vi "Main.vi"() -> (0 "error out":errorcluster)   [LabVIEW 2018]
uses:
  Controls/Cluster_HMI_VIFP - 2.ctl
  <vilib>/RAFA Solutions/Harmony UI Controls Kit/Numeric/Horizontal Progress Bar.ctl
  <vilib>/RAFA Solutions/Harmony UI Controls Kit/Numeric/Numeric Indicator.ctl
  Global/Demo.vi
  Global/Error Queue Reference.vi
  Global/datos usuario.vi
  <vilib>/addons/database/Connection.llb/DB Tools Open Connec (Path).vi
  Global/TimerReferences.vi
  Global/globalGenerador2_HMI.vi
  Global/globalGenerador3_HMI.vi
  Global/globalGenerador4_HMI.vi
  Global/globalGenerador5_HMI.vi
  Global/globalGenerador6_HMI.vi
  Global/globalGenerador1_HMI.vi
  Global/globalEventos.vi
  Global/MSG.vi
  <vilib>/addons/database/NI_Database_API.lvlib
  <vilib>/RAFA Solutions/Harmony UI Controls Kit/Flat UI Design.lvlib
panel:
  in  "type specifier VI Refnum (for type only) 16":refnum<vi>
  out "Mensaje Error":string
  in  "type specifier VI Refnum (for type only)":refnum<vi>
  in  "type specifier VI Refnum (for type only) 15":refnum<vi>
  in  "type specifier VI Refnum (for type only) 14":refnum<vi>
  in  "type specifier VI Refnum (for type only) 13":refnum<vi>
  in  "type specifier VI Refnum (for type only) 12":refnum<vi>
  in  "type specifier VI Refnum (for type only) 11":refnum<vi>
  in  "type specifier VI Refnum (for type only) 10":refnum<vi>
  in  "type specifier VI Refnum (for type only) 9":refnum<vi>
  in  "type specifier VI Refnum (for type only) 8":refnum<vi>
  in  "type specifier VI Refnum (for type only) 7":refnum<vi>
  in  "type specifier VI Refnum (for type only) 6":refnum<vi>
  in  "type specifier VI Refnum (for type only) 5":refnum<vi>
  in  "type specifier VI Refnum (for type only) 4":refnum<vi>
  in  "type specifier VI Refnum (for type only) 3":refnum<vi>
  in  "type specifier VI Refnum (for type only) 2":refnum<vi>
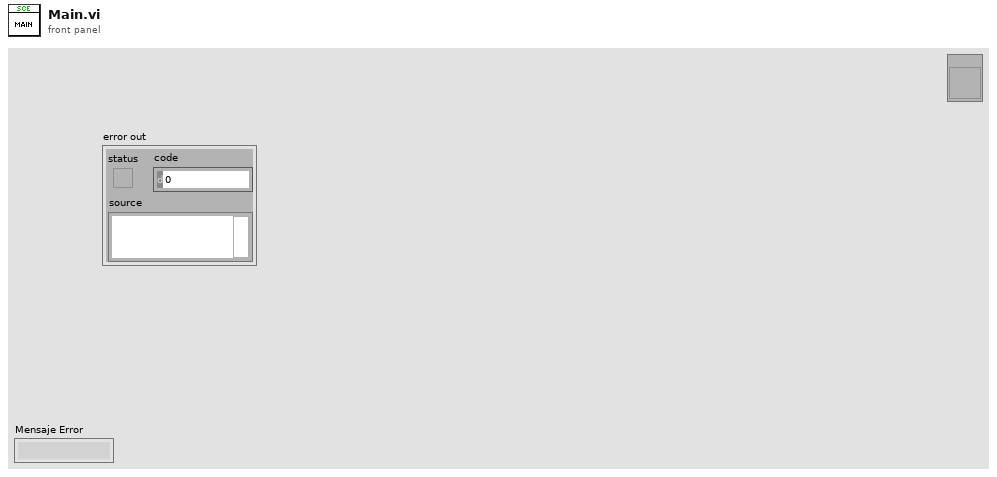
[diagram p1: front panel]
types:
  T1 = enum32{"Invalid", "Standard", "Closed", "Hidden", "Minimized", "Maximized"}
  T2 = typedef "NI_Database_API.lvlib/Conn ObjectReference.ctl" = refnum<k1>
  T3 = typedef "Equipos_Medicion_cluster.ctl" = cluster{"ID_EQUIPO":i32, "IP_EQUIPO":string, "NOMBRE_EQUIPO":string, "ESTADO_EQUIPO":string, "DESCRIPCION":string, "ID_MEDICION":i32, "ESTADO_MEDICION":string, "TIEMPO_MEDICION":string}
  T4 = typedef "Cluster_HMI_VIFP - 2.ctl" = cluster{"L2":T5, "L3":T5, "I2":T5, "I3":T5, "Frecuencia [Hz]":T6, "Potencia Total [kW]":T6, "Factor de Potencia":T6, "L1":T5, "I1":T5}
  T5 = typedef "Flat UI Design.lvlib/Horizontal Progress Bar.ctl" = sgl
  T6 = typedef "Flat UI Design.lvlib/Numeric Indicator.ctl" = sgl
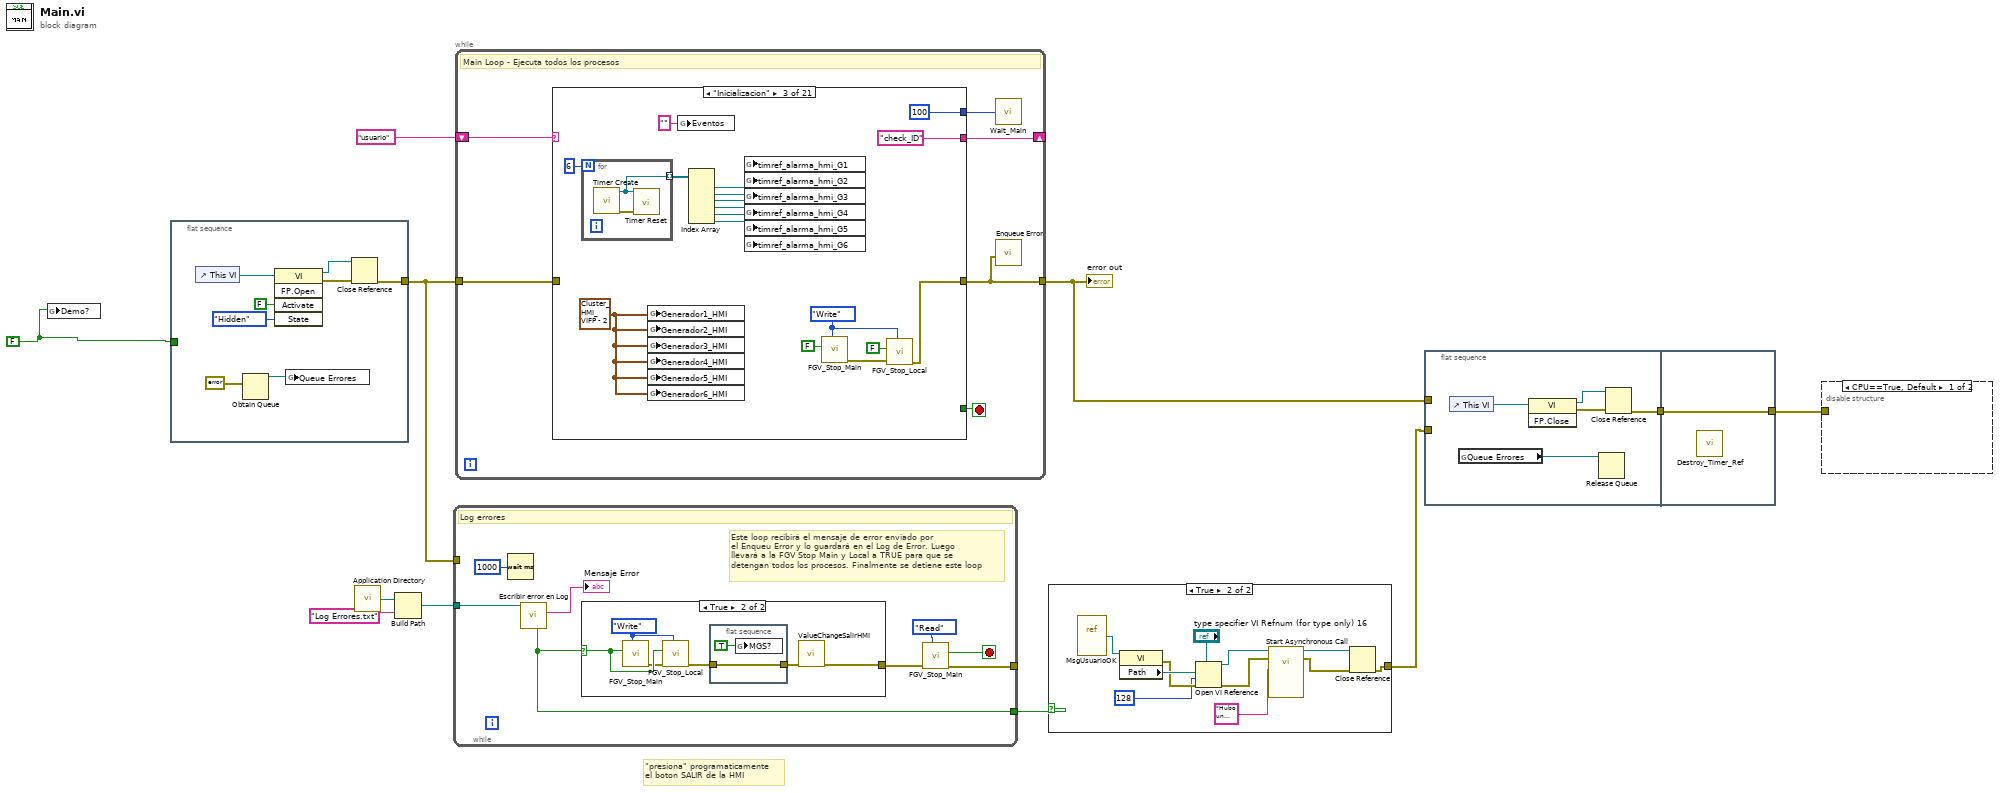
[diagram p0: block diagram]
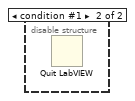
[diagram p4: hidden frame]
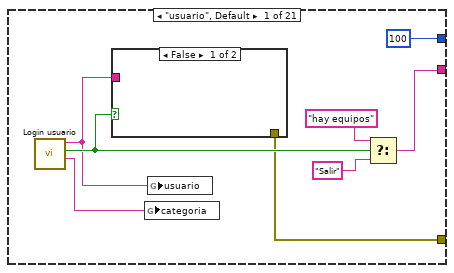
[diagram p5: hidden frame]
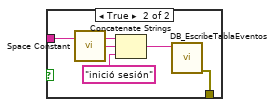
[diagram p6: hidden frame]
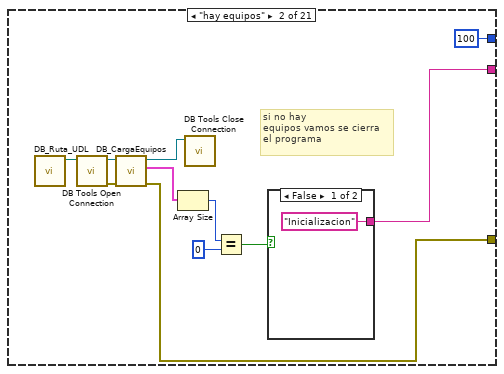
[diagram p7: hidden frame]
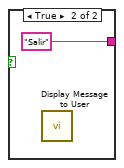
[diagram p8: hidden frame]
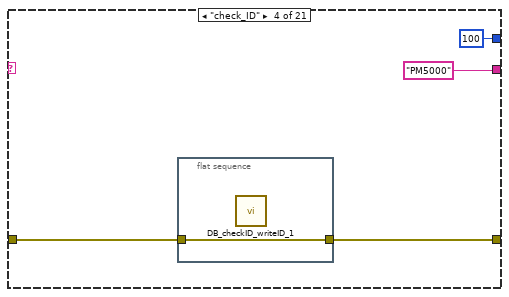
[diagram p9: hidden frame]
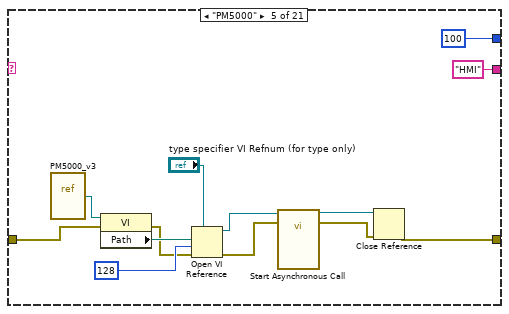
[diagram p10: hidden frame]
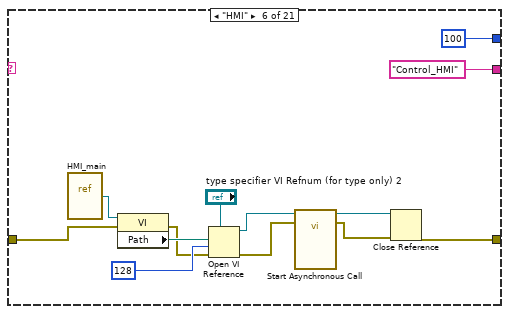
[diagram p11: hidden frame]
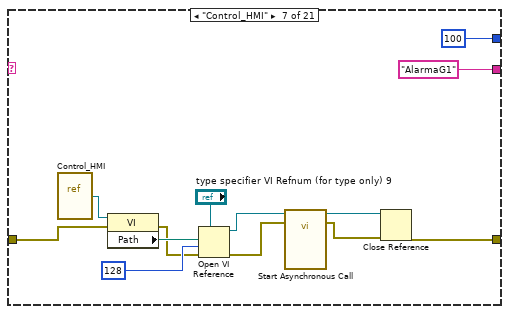
[diagram p12: hidden frame]
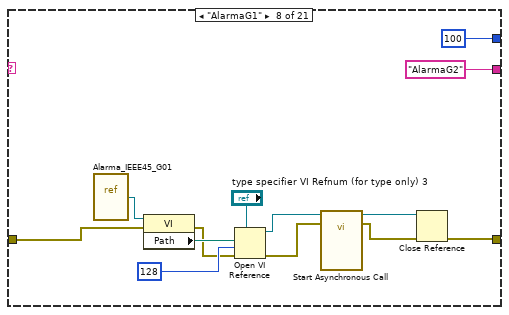
[diagram p13: hidden frame]
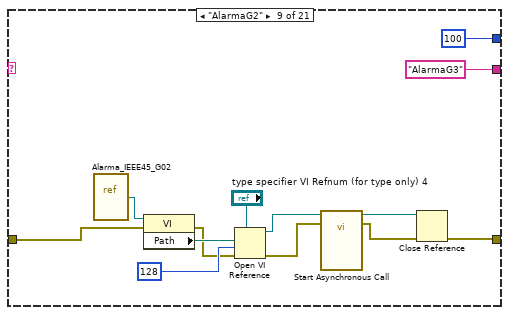
[diagram p14: hidden frame]
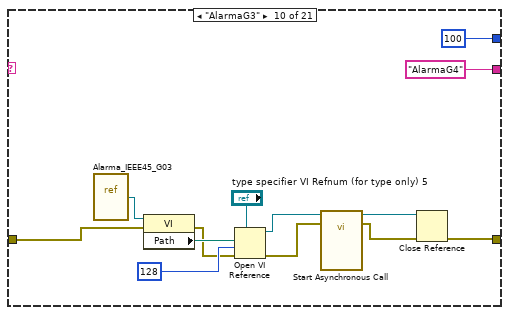
[diagram p15: hidden frame]
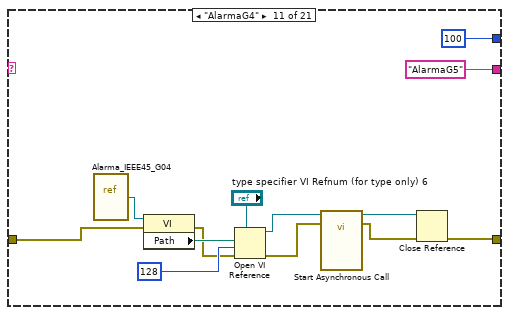
[diagram p16: hidden frame]
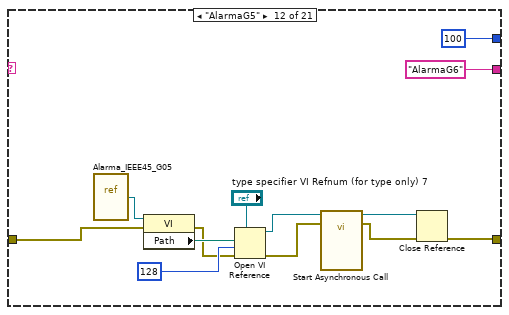
[diagram p17: hidden frame]
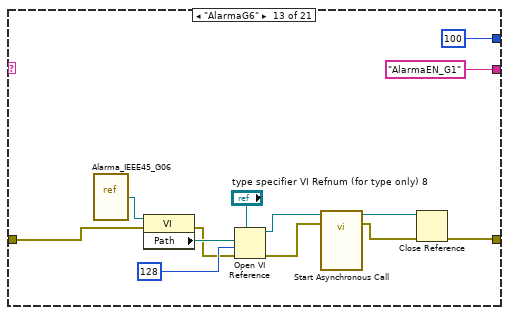
[diagram p18: hidden frame]
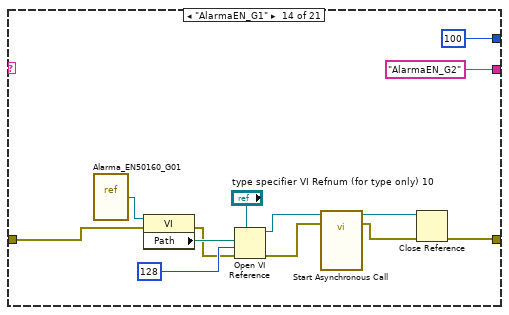
[diagram p19: hidden frame]
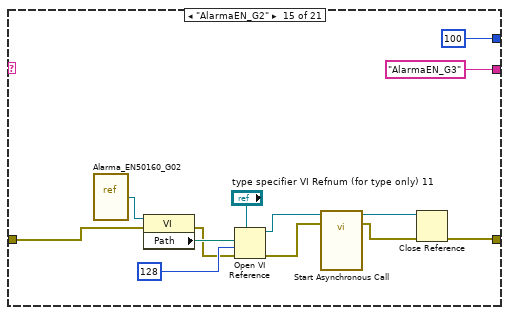
[diagram p20: hidden frame]
diagram:
  w2 = FALSE ("Demo?")
  # "\"presiona\" programaticamente\nel boton SALIR de la HMI"
  n1 = global write "Demo.vi" "Demo?"(w2) -> ()
  n2 = flat-sequence {
    tunnel: [w14] -> w7
    tunnel: w2 -> [_]
    frame #0 {
      n3 = control-ref of="This VI"() -> (w19:refnum<vi>)
      n4 = Obtain Queue(element data type=errorcluster {"status"=FALSE, "code"=0, "source"=""} ("error out")) -> (queue out=w13:refnum<queue>)  [unwired: 4 in, 2 out]
      n5 = invoke class="VI" method="FP.Open"(reference=w19, "Activate"=FALSE ("Activate?"), "State"=T1."Hidden") -> (reference out=w16:refnum<vi>, error out=w15:errorcluster)  [unwired: 2 in, 3 out]
      n6 = global write "Error Queue Reference.vi" "Queue Errores"(w13) -> ()
      n7 = Close Reference(reference=w16, error in (no error)=w15) -> (error out=w14:errorcluster)
    }
  }
  n8 = call <vilib>:"Application Directory.vi"() -> ("Application Directory"=w10:path)
  n9 = Build Path(base path=w10, name or relative path="Log Errores.txt") -> (appended path=w8:path)
  n10 = while {
    tunnel: w8 -> [w27]
    tunnel: w7 -> [_]
    tunnel: [w22] -> _
    tunnel: [w20] -> w6
    stop <- w23 stop-if-true
    # "Este loop recibirá el mensaje de error enviado por \nel Enqueu Error y lo guardará en el Log de Error. Luego\nllevará a la FGV Stop Main y Local a TRUE para que se\ndetengan todos los procesos. Finalmente se detiene este loop"
    # "Log errores"
    n11 = Wait (ms)(milliseconds to wait=u32 1000) -> ()  [unwired: 1 out]
    n12 = call "Escribir error en Log.vi"("Ruta Log"=w27) -> ("Mensaje Error"=→"Mensaje Error":string, "error"=w20:bool)  [unwired: 6 in, 3 out]
    n13 = case shown="True" w20 {
      selector: w20 -> [_ w32]
      tunnel: [_ w28] -> w21
      frame False {
      }
      frame True {
        w33 = enum16{"Read", "Write"}."Write" ("Action")
        n14 = call "FGV_Stop_Main.vi"("Action"=w33, "Var In"=w32) -> ("Error Out"=w31:errorcluster)  [unwired: 8 in, 1 out]
        n15 = call "FGV_Stop_Local.vi"("Action"=w33, "Error In (no error)"=w31, "Var In"=w32) -> ("Error Out"=w30:errorcluster)  [unwired: 7 in, 1 out]
        n16 = flat-sequence {
          tunnel: w30 -> [w34]
          tunnel: [w34] -> w29
          frame #0 {
            n17 = global write "MSG.vi" "MGS?"(TRUE ("MGS?")) -> ()
          }
        }
        n18 = call "ValueChangeSalirHMI.vi"("error in (no error)"=w29) -> ("error out"=w28:errorcluster)  [unwired: 10 in]
      }
    }
    n19 = call "FGV_Stop_Main.vi"("Action"=enum16{"Read", "Write"}."Read", "Error In (no error)"=w21) -> ("Error Out"=w22:errorcluster, "Var Out"=w23:bool)  [unwired: 8 in]
  }
  n20 = while {
    shift-right: [w40] -> _
    shift-left: "usuario" -> [w41]
    tunnel: w7 -> [w37]
    tunnel: [w36] -> w5
    stop <- w39 stop-if-true
    # "Main Loop - Ejecuta todos los procesos"
    n21 = case shown="\"Inicializacion\"" w41 {
      tunnel: [w46 w61 "check_ID" "PM5000" "HMI" "Control_HMI" "AlarmaG1" "AlarmaG2" "AlarmaG3" "AlarmaG4" "AlarmaG5" "AlarmaG6" "AlarmaEN_G1" "AlarmaEN_G2" "AlarmaEN_G3" "AlarmaEN_G4" "AlarmaEN_G5" "AlarmaEN_G6" "Idle" w289 ""] -> w40
      tunnel: [_ _ _ _ _ _ _ _ _ _ _ _ _ _ _ _ _ _ _ _ TRUE] -> w39
      tunnel: [u32 100 ("Wait time (msec)") u32 100 ("Wait time (msec)") u32 100 ("Wait time (msec)") u32 100 ("Wait time (msec)") u32 100 ("Wait time (msec)") u32 100 ("Wait time (msec)") u32 100 ("Wait time (msec)") u32 100 ("Wait time (msec)") u32 100 ("Wait time (msec)") u32 100 ("Wait time (msec)") u32 100 ("Wait time (msec)") u32 100 ("Wait time (msec)") u32 100 ("Wait time (msec)") u32 100 ("Wait time (msec)") u32 100 ("Wait time (msec)") u32 100 ("Wait time (msec)") u32 100 ("Wait time (msec)") u32 100 ("Wait time (msec)") u32 100 ("Wait time (msec)") u32 1000 ("Wait time (msec)") u32 100 ("Wait time (msec)")] -> w38
      tunnel: w37 -> [_ _ _ w88 w95 w106 w121 w132 w145 w158 w171 w184 w197 w210 w223 w236 w249 w262 w275 _ w294]
      tunnel: [w42 w56 w69 w87 w103 w105 w120 w131 w144 w157 w170 w183 w196 w209 w222 w235 w248 w261 w274 w287 w294] -> w36
      frame "usuario", Default {
        n22 = call "Login usuario.vi"() -> ("categoria out"=w43:string, "Usuario y Pass OK?"=w45:bool, "Usuario out"=w44:string)  [unwired: 9 in]
        n23 = case shown="False" w45 {
          tunnel: w44 -> [_ w54]
          tunnel: [_ w50] -> w42
          frame False {
          }
          frame True {
            n24 = call <vilib>:"Space Constant.vi"() -> ("String"=w53:string)
            n25 = Concatenate Strings(w54, w53, "inició sesión" ("string")) -> (w51:string)
            n26 = call "DB_EscribeTablaEventos.vi"("DESCRIPCION"=w51) -> ("error out"=w50:errorcluster)  [unwired: 10 in]
          }
        }
        n27 = global write "datos usuario.vi" "categoria"(w43) -> ()
        n28 = global write "datos usuario.vi" "usuario"(w44) -> ()
        n29 = Select(t="hay equipos", s=w45, f="Salir") -> (s? t:f=w46:string)
      }
      frame "hay equipos" {
        # "si no hay \nequipos vamos se cierra \nel programa"
        n30 = call "DB_Ruta_UDL.vi"() -> ("UDL ruta"=w57:path)  [unwired: 11 in]
        n31 = call-poly <vilib>:"DB Tools Open Connection.vi"("connection information"=w57) -> ("error out"=w59:errorcluster, "connection reference"=w58:T2)  [unwired: 7 in]
        n32 = call "DB_CargaEquipos.vi"("error in (no error)"=w59, "db in"=w58) -> ("error out"=w56:errorcluster, "Equipos_out"=w63:T3[], "db out"=w55:T2)  [unwired: 2 in, 5 out]
        n33 = Array Size(array=w63) -> (size(s)=w65:i32)
        n34 = call <vilib>:"DB Tools Close Connection.vi"("connection reference"=w55) -> ()  [unwired: 6 in, 1 out]
        n35 = Equal?(x=w65, y=0) -> (x = y?=w62:bool)
        n36 = case shown="False" w62 {
          tunnel: ["Inicializacion" "Salir"] -> w61
          frame False {
          }
          frame True {
            n37 = call "Display Message to User"() -> ()  [unwired: 10 in, 2 out]
          }
        }
      }
      frame "Inicializacion" {
        w70 = T4 {"L2"=0.0, "L3"=0.0, "I2"=0.0, "I3"=0.0, "Frecuencia [Hz]"=0.0, "Potencia Total [kW]"=0.0, "Factor de Potencia"=0.0, "L1"=0.0, "I1"=0.0} ("Generador1_HMI")
        w81 = enum16{"Read", "Write"}."Write" ("Action")
        n38 = for {
          N: 6 -> [_]
          tunnel: [w85] -> w78 mode=indexing
          n39 = call "Timer Create.vi"() -> ("error out"=w86:errorcluster, "Timer reference out"=w85:refnum<data-value>)  [unwired: 10 in]
          n40 = call "Timer Reset.vi"("error in (no error)"=w86, "Timer reference"=w85) -> ()  [unwired: 8 in, 2 out]
        }
        n41 = global write "globalGenerador1_HMI.vi" "Generador1_HMI"(w70) -> ()
        n42 = global write "globalGenerador2_HMI.vi" "Generador2_HMI"(w70) -> ()
        n43 = global write "globalGenerador3_HMI.vi" "Generador3_HMI"(w70) -> ()
        n44 = global write "globalGenerador4_HMI.vi" "Generador4_HMI"(w70) -> ()
        n45 = global write "globalGenerador5_HMI.vi" "Generador5_HMI"(w70) -> ()
        n46 = global write "globalGenerador6_HMI.vi" "Generador6_HMI"(w70) -> ()
        n47 = global write "globalEventos.vi" "Eventos"("" ("Eventos")) -> ()
        n48 = Index Array(array=w78) -> (element #1=w77:refnum<data-value>, element #2=w76:refnum<data-value>, element #3=w75:refnum<data-value>, element #4=w74:refnum<data-value>, element #5=w73:refnum<data-value>, element #6=w72:refnum<data-value>)  [unwired: 6 in]
        n49 = global write "TimerReferences.vi" "timref_alarma_hmi_G1"(w77) -> ()
        n50 = global write "TimerReferences.vi" "timref_alarma_hmi_G2"(w76) -> ()
        n51 = global write "TimerReferences.vi" "timref_alarma_hmi_G3"(w75) -> ()
        n52 = global write "TimerReferences.vi" "timref_alarma_hmi_G4"(w74) -> ()
        n53 = global write "TimerReferences.vi" "timref_alarma_hmi_G5"(w73) -> ()
        n54 = global write "TimerReferences.vi" "timref_alarma_hmi_G6"(w72) -> ()
        n55 = call "FGV_Stop_Main.vi"("Action"=w81, "Var In"=FALSE) -> ("Error Out"=w82:errorcluster)  [unwired: 8 in, 1 out]
        n56 = call "FGV_Stop_Local.vi"("Action"=w81, "Error In (no error)"=w82, "Var In"=FALSE) -> ("Error Out"=w69:errorcluster)  [unwired: 7 in, 1 out]
      }
      frame "check_ID" {
        n57 = flat-sequence {
          tunnel: w88 -> [w91]
          tunnel: [w91] -> w87
          frame #0 {
            n58 = call "DB_checkID_writeID_1.vi"() -> ()  [unwired: 12 in]
          }
        }
      }
      frame "PM5000" {
        n59 = vi-ref "PM5000_v3.vi"() -> (w97:refnum<vi>)
        n60 = property class="VI"(reference=w97, error in=w95) -> (error out=w94:errorcluster, "Path"=w96:path)  [unwired: 1 out]
        n61 = Open VI Reference(type specifier VI Refnum (for type only)="type specifier VI Refnum (for type only)", vi path=w96, options=128, error in (no error)=w94) -> (vi reference=w99:refnum<vi>, error out=w102:errorcluster)  [unwired: 2 in]
        n62 = call-by-ref "Start Asynchronous Call"(reference=w99, error in=w102) -> (reference out=w101:refnum<vi>, error out=w100:errorcluster)  [unwired: 12 in]
        n63 = Close Reference(reference=w101, error in (no error)=w100) -> (error out=w103:errorcluster)
      }
      frame "HMI" {
        n64 = vi-ref "HMI_main.vi"() -> (w109:refnum<vi>)
        n65 = property class="VI"(reference=w109, error in=w106) -> (error out=w107:errorcluster, "Path"=w108:path)  [unwired: 1 out]
        n66 = Open VI Reference(type specifier VI Refnum (for type only)="type specifier VI Refnum (for type only) 2", vi path=w108, options=128, error in (no error)=w107) -> (vi reference=w111:refnum<vi>, error out=w115:errorcluster)  [unwired: 2 in]
        n67 = call-by-ref "Start Asynchronous Call"(reference=w111, error in=w115) -> (reference out=w114:refnum<vi>, error out=w113:errorcluster)  [unwired: 12 in]
        n68 = Close Reference(reference=w114, error in (no error)=w113) -> (error out=w105:errorcluster)
      }
      frame "Control_HMI" {
        n69 = vi-ref "Control_HMI.vi"() -> (w124:refnum<vi>)
        n70 = property class="VI"(reference=w124, error in=w121) -> (error out=w122:errorcluster, "Path"=w123:path)  [unwired: 1 out]
        n71 = Open VI Reference(type specifier VI Refnum (for type only)="type specifier VI Refnum (for type only) 9", vi path=w123, options=128, error in (no error)=w122) -> (vi reference=w126:refnum<vi>, error out=w130:errorcluster)  [unwired: 2 in]
        n72 = call-by-ref "Start Asynchronous Call"(reference=w126, error in=w130) -> (reference out=w129:refnum<vi>, error out=w128:errorcluster)  [unwired: 12 in]
        n73 = Close Reference(reference=w129, error in (no error)=w128) -> (error out=w120:errorcluster)
      }
      frame "AlarmaG1" {
        n74 = vi-ref "Alarma_IEEE45_G01.vi"() -> (w135:refnum<vi>)
        n75 = property class="VI"(reference=w135, error in=w132) -> (error out=w133:errorcluster, "Path"=w134:path)  [unwired: 1 out]
        n76 = Open VI Reference(type specifier VI Refnum (for type only)="type specifier VI Refnum (for type only) 3", vi path=w134, options=128, error in (no error)=w133) -> (vi reference=w137:refnum<vi>, error out=w141:errorcluster)  [unwired: 2 in]
        n77 = call-by-ref "Start Asynchronous Call"(reference=w137, error in=w141) -> (reference out=w140:refnum<vi>, error out=w139:errorcluster)  [unwired: 11 in, 1 out]
        n78 = Close Reference(reference=w140, error in (no error)=w139) -> (error out=w131:errorcluster)
      }
      frame "AlarmaG2" {
        n79 = vi-ref "Alarma_IEEE45_G02.vi"() -> (w148:refnum<vi>)
        n80 = property class="VI"(reference=w148, error in=w145) -> (error out=w146:errorcluster, "Path"=w147:path)  [unwired: 1 out]
        n81 = Open VI Reference(type specifier VI Refnum (for type only)="type specifier VI Refnum (for type only) 4", vi path=w147, options=128, error in (no error)=w146) -> (vi reference=w150:refnum<vi>, error out=w154:errorcluster)  [unwired: 2 in]
        n82 = call-by-ref "Start Asynchronous Call"(reference=w150, error in=w154) -> (reference out=w153:refnum<vi>, error out=w152:errorcluster)  [unwired: 11 in, 1 out]
        n83 = Close Reference(reference=w153, error in (no error)=w152) -> (error out=w144:errorcluster)
      }
      frame "AlarmaG3" {
        n84 = vi-ref "Alarma_IEEE45_G03.vi"() -> (w161:refnum<vi>)
        n85 = property class="VI"(reference=w161, error in=w158) -> (error out=w159:errorcluster, "Path"=w160:path)  [unwired: 1 out]
        n86 = Open VI Reference(type specifier VI Refnum (for type only)="type specifier VI Refnum (for type only) 5", vi path=w160, options=128, error in (no error)=w159) -> (vi reference=w163:refnum<vi>, error out=w167:errorcluster)  [unwired: 2 in]
        n87 = call-by-ref "Start Asynchronous Call"(reference=w163, error in=w167) -> (reference out=w166:refnum<vi>, error out=w165:errorcluster)  [unwired: 11 in, 1 out]
        n88 = Close Reference(reference=w166, error in (no error)=w165) -> (error out=w157:errorcluster)
      }
      frame "AlarmaG4" {
        n89 = vi-ref "Alarma_IEEE45_G04.vi"() -> (w174:refnum<vi>)
        n90 = property class="VI"(reference=w174, error in=w171) -> (error out=w172:errorcluster, "Path"=w173:path)  [unwired: 1 out]
        n91 = Open VI Reference(type specifier VI Refnum (for type only)="type specifier VI Refnum (for type only) 6", vi path=w173, options=128, error in (no error)=w172) -> (vi reference=w176:refnum<vi>, error out=w180:errorcluster)  [unwired: 2 in]
        n92 = call-by-ref "Start Asynchronous Call"(reference=w176, error in=w180) -> (reference out=w179:refnum<vi>, error out=w178:errorcluster)  [unwired: 11 in, 1 out]
        n93 = Close Reference(reference=w179, error in (no error)=w178) -> (error out=w170:errorcluster)
      }
      frame "AlarmaG5" {
        n94 = vi-ref "Alarma_IEEE45_G05.vi"() -> (w187:refnum<vi>)
        n95 = property class="VI"(reference=w187, error in=w184) -> (error out=w185:errorcluster, "Path"=w186:path)  [unwired: 1 out]
        n96 = Open VI Reference(type specifier VI Refnum (for type only)="type specifier VI Refnum (for type only) 7", vi path=w186, options=128, error in (no error)=w185) -> (vi reference=w189:refnum<vi>, error out=w193:errorcluster)  [unwired: 2 in]
        n97 = call-by-ref "Start Asynchronous Call"(reference=w189, error in=w193) -> (reference out=w192:refnum<vi>, error out=w191:errorcluster)  [unwired: 11 in, 1 out]
        n98 = Close Reference(reference=w192, error in (no error)=w191) -> (error out=w183:errorcluster)
      }
      frame "AlarmaG6" {
        n99 = vi-ref "Alarma_IEEE45_G06.vi"() -> (w200:refnum<vi>)
        n100 = property class="VI"(reference=w200, error in=w197) -> (error out=w198:errorcluster, "Path"=w199:path)  [unwired: 1 out]
        n101 = Open VI Reference(type specifier VI Refnum (for type only)="type specifier VI Refnum (for type only) 8", vi path=w199, options=128, error in (no error)=w198) -> (vi reference=w202:refnum<vi>, error out=w206:errorcluster)  [unwired: 2 in]
        n102 = call-by-ref "Start Asynchronous Call"(reference=w202, error in=w206) -> (reference out=w205:refnum<vi>, error out=w204:errorcluster)  [unwired: 11 in, 1 out]
        n103 = Close Reference(reference=w205, error in (no error)=w204) -> (error out=w196:errorcluster)
      }
      frame "AlarmaEN_G1" {
        n104 = vi-ref "Alarma_EN50160_G01.vi"() -> (w213:refnum<vi>)
        n105 = property class="VI"(reference=w213, error in=w210) -> (error out=w211:errorcluster, "Path"=w212:path)  [unwired: 1 out]
        n106 = Open VI Reference(type specifier VI Refnum (for type only)="type specifier VI Refnum (for type only) 10", vi path=w212, options=128, error in (no error)=w211) -> (vi reference=w215:refnum<vi>, error out=w219:errorcluster)  [unwired: 2 in]
        n107 = call-by-ref "Start Asynchronous Call"(reference=w215, error in=w219) -> (reference out=w218:refnum<vi>, error out=w217:errorcluster)  [unwired: 12 in]
        n108 = Close Reference(reference=w218, error in (no error)=w217) -> (error out=w209:errorcluster)
      }
      frame "AlarmaEN_G2" {
        n109 = vi-ref "Alarma_EN50160_G02.vi"() -> (w226:refnum<vi>)
        n110 = property class="VI"(reference=w226, error in=w223) -> (error out=w224:errorcluster, "Path"=w225:path)  [unwired: 1 out]
        n111 = Open VI Reference(type specifier VI Refnum (for type only)="type specifier VI Refnum (for type only) 11", vi path=w225, options=128, error in (no error)=w224) -> (vi reference=w228:refnum<vi>, error out=w232:errorcluster)  [unwired: 2 in]
        n112 = call-by-ref "Start Asynchronous Call"(reference=w228, error in=w232) -> (reference out=w231:refnum<vi>, error out=w230:errorcluster)  [unwired: 12 in]
        n113 = Close Reference(reference=w231, error in (no error)=w230) -> (error out=w222:errorcluster)
      }
      frame "AlarmaEN_G3" {
        n114 = vi-ref "Alarma_EN50160_G03.vi"() -> (w239:refnum<vi>)
        n115 = property class="VI"(reference=w239, error in=w236) -> (error out=w237:errorcluster, "Path"=w238:path)  [unwired: 1 out]
        n116 = Open VI Reference(type specifier VI Refnum (for type only)="type specifier VI Refnum (for type only) 12", vi path=w238, options=128, error in (no error)=w237) -> (vi reference=w241:refnum<vi>, error out=w245:errorcluster)  [unwired: 2 in]
        n117 = call-by-ref "Start Asynchronous Call"(reference=w241, error in=w245) -> (reference out=w244:refnum<vi>, error out=w243:errorcluster)  [unwired: 12 in]
        n118 = Close Reference(reference=w244, error in (no error)=w243) -> (error out=w235:errorcluster)
      }
      frame "AlarmaEN_G4" {
        n119 = vi-ref "Alarma_EN50160_G04.vi"() -> (w252:refnum<vi>)
        n120 = property class="VI"(reference=w252, error in=w249) -> (error out=w250:errorcluster, "Path"=w251:path)  [unwired: 1 out]
        n121 = Open VI Reference(type specifier VI Refnum (for type only)="type specifier VI Refnum (for type only) 13", vi path=w251, options=128, error in (no error)=w250) -> (vi reference=w254:refnum<vi>, error out=w258:errorcluster)  [unwired: 2 in]
        n122 = call-by-ref "Start Asynchronous Call"(reference=w254, error in=w258) -> (reference out=w257:refnum<vi>, error out=w256:errorcluster)  [unwired: 12 in]
        n123 = Close Reference(reference=w257, error in (no error)=w256) -> (error out=w248:errorcluster)
      }
      frame "AlarmaEN_G5" {
        n124 = vi-ref "Alarma_EN50160_G05.vi"() -> (w265:refnum<vi>)
        n125 = property class="VI"(reference=w265, error in=w262) -> (error out=w263:errorcluster, "Path"=w264:path)  [unwired: 1 out]
        n126 = Open VI Reference(type specifier VI Refnum (for type only)="type specifier VI Refnum (for type only) 14", vi path=w264, options=128, error in (no error)=w263) -> (vi reference=w267:refnum<vi>, error out=w271:errorcluster)  [unwired: 2 in]
        n127 = call-by-ref "Start Asynchronous Call"(reference=w267, error in=w271) -> (reference out=w270:refnum<vi>, error out=w269:errorcluster)  [unwired: 12 in]
        n128 = Close Reference(reference=w270, error in (no error)=w269) -> (error out=w261:errorcluster)
      }
      frame "AlarmaEN_G6" {
        n129 = vi-ref "Alarma_EN50160_G06.vi"() -> (w278:refnum<vi>)
        n130 = property class="VI"(reference=w278, error in=w275) -> (error out=w276:errorcluster, "Path"=w277:path)  [unwired: 1 out]
        n131 = Open VI Reference(type specifier VI Refnum (for type only)="type specifier VI Refnum (for type only) 15", vi path=w277, options=128, error in (no error)=w276) -> (vi reference=w280:refnum<vi>, error out=w284:errorcluster)  [unwired: 2 in]
        n132 = call-by-ref "Start Asynchronous Call"(reference=w280, error in=w284) -> (reference out=w283:refnum<vi>, error out=w282:errorcluster)  [unwired: 12 in]
        n133 = Close Reference(reference=w283, error in (no error)=w282) -> (error out=w274:errorcluster)
      }
      frame "Idle" {
        n134 = call "FGV_Stop_Main.vi"("Action"=enum16{"Read", "Write"}."Read") -> ("Error Out"=w287:errorcluster, "Var Out"=w292:bool)  [unwired: 9 in]
        n135 = Select(t="Salir", s=w292, f="Idle") -> (s? t:f=w289:string)
      }
      frame "Salir" {
      }
    }
    n136 = call "Wait_Main.vi"("Wait time (msec)"=w38) -> ()  [unwired: 5 in]
    n137 = call "Enqueue Error.vi"("error in"=w36) -> ()  [unwired: 9 in, 2 out]
  }
  "error out" <- w5
  n138 = case shown="True" w6 {
    tunnel: [_ w298] -> w4
    frame False {
    }
    frame True {
      n139 = vi-ref "MsgUsuarioOK.vi"() -> (w303:refnum<vi>)
      n140 = property class="VI"(reference=w303) -> (error out=w301:errorcluster, "Path"=w302:path)  [unwired: 1 in, 1 out]
      n141 = Open VI Reference(type specifier VI Refnum (for type only)="type specifier VI Refnum (for type only) 16", vi path=w302, options=128, error in (no error)=w301) -> (vi reference=w304:refnum<vi>, error out=w308:errorcluster)  [unwired: 2 in]
      n142 = call-by-ref "Start Asynchronous Call"(reference=w304, error in=w308, "texto"="Hubo un error de sistema y se cerrará la aplicación. Revise el archivo \"Log Errores.txt\" para conocer el motivo del error. Si el error continua, póngase en contacto con el administrador de la aplicación.") -> (reference out=w307:refnum<vi>, error out=w306:errorcluster)  [unwired: 10 in, 1 out]
      n143 = Close Reference(reference=w307, error in (no error)=w306) -> (error out=w298:errorcluster)
    }
  }
  n144 = flat-sequence {
    tunnel: w5 -> [_]
    tunnel: w4 -> [_]
    tunnel: [w310] -> w1
    tunnel: [w314] -> w3
    tunnel: w1 -> [w314]
    frame #0 {
      n145 = control-ref of="This VI"() -> (w313:refnum<vi>)
      n146 = global read "Error Queue Reference.vi" "Queue Errores"() -> (w309:refnum<queue>)
      n147 = invoke class="VI" method="FP.Close"(reference=w313) -> (reference out=w312:refnum<vi>, error out=w311:errorcluster)  [unwired: 2 in, 1 out]
      n148 = Release Queue(queue=w309) -> ()  [unwired: 2 in, 3 out]
      n149 = Close Reference(reference=w312, error in (no error)=w311) -> (error out=w310:errorcluster)
    }
    frame #1 {
      n150 = call "Destroy_Timer_Ref.vi"() -> ()  [unwired: 12 in]
    }
  }
  n151 = disable-structure shown="CPU==True, Default" {
    disable-tunnel: w3 -> [_ _]
    frame condition #0 (active) {
    }
    frame condition #1 {
      n152 = Quit LabVIEW() -> ()  [unwired: 1 in]
    }
  }
